vi "user32_SwitchToThisWindow.vi"(7 "fAltTab(F)":bool, 8 "错误输入（无错误）":errorcluster, 11 "hWnd":u32) -> (0 "错误输出":errorcluster, 3 "dup hWnd":u32)   [LabVIEW 2011]
doc: "该函数将焦点切换指定的窗口，并将其带到前台。"
uses:
  user32.dll
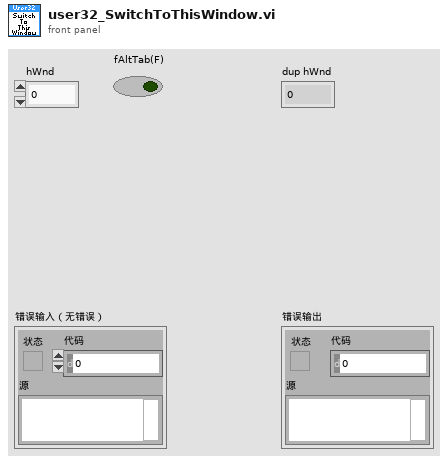
[diagram p1: front panel]
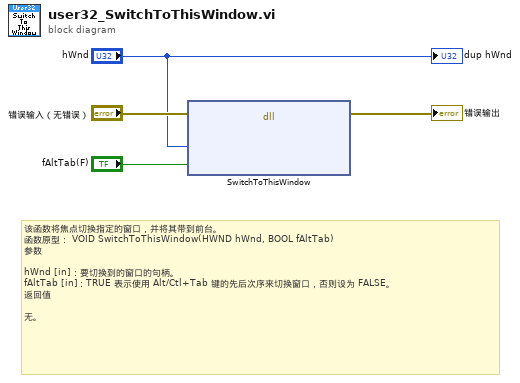
[diagram p0: block diagram]
diagram:
  # "该函数将焦点切换指定的窗口，并将其带到前台。\n函数原型： VOID SwitchToThisWindow(HWND hWnd, BOOL fAltTab)\n参数\n\nhWnd [in]：要切换到的窗口的句柄。\nfAltTab [in]：TRUE 表示使用 Alt/Ctl+Tab 键的先后次序来切换窗口，否则设为 FALSE。\n返回值\n\n无。"
  n1 = dll-call lib="user32.dll" fn="SwitchToThisWindow"(error in="错误输入（无错误）", "hWnd"="hWnd", "fAltTab"="fAltTab(F)") -> (error out=→"错误输出":errorcluster)  [unwired: 5 in, 1 out]
  "dup hWnd" <- "hWnd"
